vi "0037-Sub_GPIO_1ON.vi"(8 "エラー出力 2":errorcluster caption="エラー入力", 9 "ブール":bool, 10 "GPIO":u8, 11 "device":i32) -> (0 "エラー出力":errorcluster, 3 "deviceOut":T1)   [LabVIEW 2014]
uses:
  LV-CP2112_2014/LVProject/private/CP2112_device.ctl
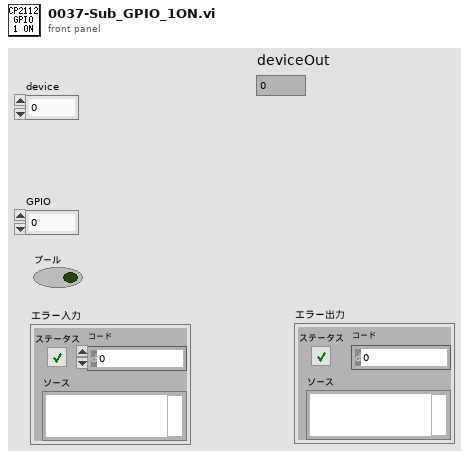
[diagram p1: front panel]
types:
  T1 = typedef "CP2112_device.ctl" = i32
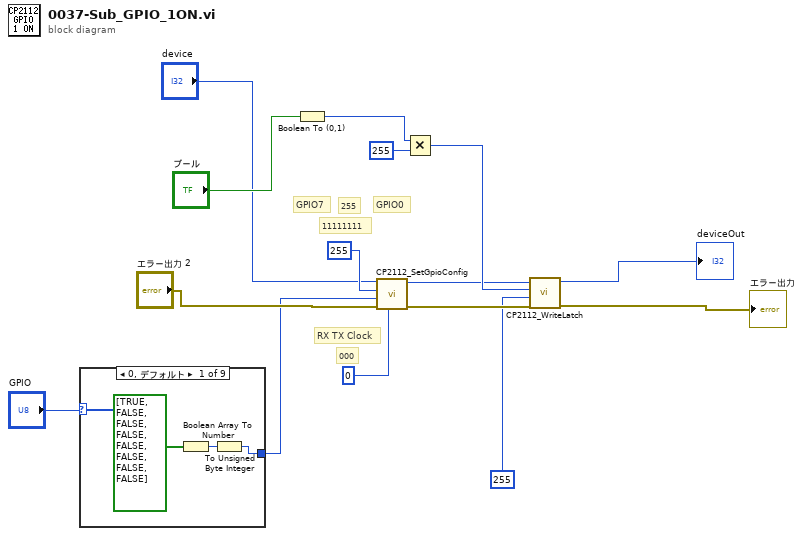
[diagram p0: block diagram]
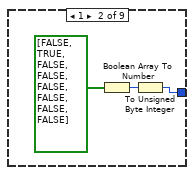
[diagram p2: hidden frame]
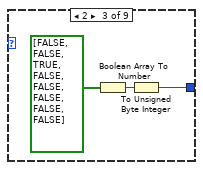
[diagram p3: hidden frame]
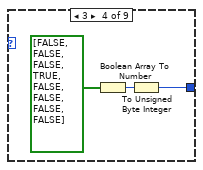
[diagram p4: hidden frame]
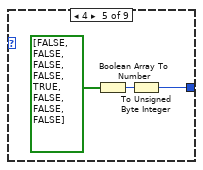
[diagram p5: hidden frame]
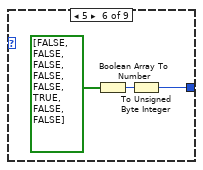
[diagram p6: hidden frame]
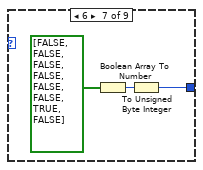
[diagram p7: hidden frame]
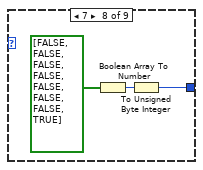
[diagram p8: hidden frame]
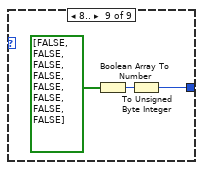
[diagram p9: hidden frame]
diagram:
  # "255"
  # "RX TX Clock"
  # "GPIO7"
  # "GPIO0"
  # "000"
  # "11111111"
  n1 = case shown="0, デフォルト" "GPIO" {
    tunnel: [w16 w19 w22 w25 w28 w31 w34 w37 w40] -> w1
    frame 0, Default {
      n2 = Boolean Array To Number(Boolean array=bool[] [TRUE, FALSE, FALSE, FALSE, FALSE, FALSE, FALSE, FALSE] ("ブール配列")) -> (number=w18:u32)
      n3 = To Unsigned Byte Integer(number=w18) -> (unsigned 8bit integer=w16:u8)
    }
    frame 1 {
      n4 = Boolean Array To Number(Boolean array=bool[] [FALSE, TRUE, FALSE, FALSE, FALSE, FALSE, FALSE, FALSE] ("ブール配列")) -> (number=w21:u32)
      n5 = To Unsigned Byte Integer(number=w21) -> (unsigned 8bit integer=w19:u8)
    }
    frame 2 {
      n6 = Boolean Array To Number(Boolean array=bool[] [FALSE, FALSE, TRUE, FALSE, FALSE, FALSE, FALSE, FALSE] ("ブール配列")) -> (number=w24:u32)
      n7 = To Unsigned Byte Integer(number=w24) -> (unsigned 8bit integer=w22:u8)
    }
    frame 3 {
      n8 = Boolean Array To Number(Boolean array=bool[] [FALSE, FALSE, FALSE, TRUE, FALSE, FALSE, FALSE, FALSE] ("ブール配列")) -> (number=w27:u32)
      n9 = To Unsigned Byte Integer(number=w27) -> (unsigned 8bit integer=w25:u8)
    }
    frame 4 {
      n10 = Boolean Array To Number(Boolean array=bool[] [FALSE, FALSE, FALSE, FALSE, TRUE, FALSE, FALSE, FALSE] ("ブール配列")) -> (number=w30:u32)
      n11 = To Unsigned Byte Integer(number=w30) -> (unsigned 8bit integer=w28:u8)
    }
    frame 5 {
      n12 = Boolean Array To Number(Boolean array=bool[] [FALSE, FALSE, FALSE, FALSE, FALSE, TRUE, FALSE, FALSE] ("ブール配列")) -> (number=w33:u32)
      n13 = To Unsigned Byte Integer(number=w33) -> (unsigned 8bit integer=w31:u8)
    }
    frame 6 {
      n14 = Boolean Array To Number(Boolean array=bool[] [FALSE, FALSE, FALSE, FALSE, FALSE, FALSE, TRUE, FALSE] ("ブール配列")) -> (number=w36:u32)
      n15 = To Unsigned Byte Integer(number=w36) -> (unsigned 8bit integer=w34:u8)
    }
    frame 7 {
      n16 = Boolean Array To Number(Boolean array=bool[] [FALSE, FALSE, FALSE, FALSE, FALSE, FALSE, FALSE, TRUE] ("ブール配列")) -> (number=w39:u32)
      n17 = To Unsigned Byte Integer(number=w39) -> (unsigned 8bit integer=w37:u8)
    }
    frame 8.. {
      n18 = Boolean Array To Number(Boolean array=bool[] [FALSE, FALSE, FALSE, FALSE, FALSE, FALSE, FALSE, FALSE] ("ブール配列")) -> (number=w42:u32)
      n19 = To Unsigned Byte Integer(number=w42) -> (unsigned 8bit integer=w40:u8)
    }
  }
  n20 = Boolean To (0,1)(Boolean="ブール") -> (0, 1=w12:i16)
  n21 = call "CP2112_SetGpioConfig.vi"("special"=u8 0, "error in (no error)"="エラー出力 2", "mode"=w1, "direction"=u8 255, "device"="device") -> ("error out"=w8:errorcluster, "deviceOut"=w9:T1)  [unwired: 4 in, 1 out]
  n22 = Multiply(x=w12, y=i16 255) -> (x*y=w14:i16)
  n23 = call "CP2112_WriteLatch.vi"("error in (no error)"=w8, "latchMask"=u8 255, "latchValue"=w14, "device"=w9) -> ("error out"=→"エラー出力":errorcluster, "deviceOut"=→"deviceOut":T1)  [unwired: 5 in, 1 out]
